vi "Error Name.vi"(10 "PCB LOCK":T1, 11 "Error Name":string[](array[string])=["Key Paid1(AI0)", "Key Paid1(AI1)", "Key Paid1(AI09)", "Key Paid1(AI10)", "Key Paid1(AI11)", "Key Paid1(AI12)"]) -> (3 "Error Message":string)   [LabVIEW 2015]
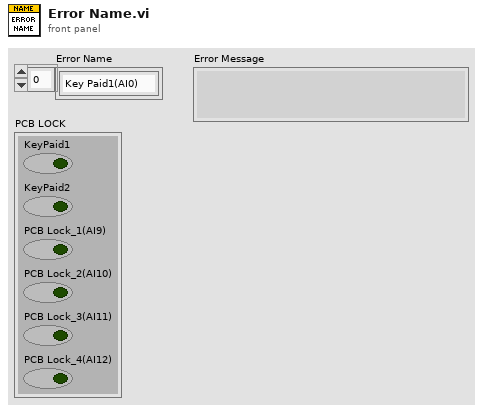
[diagram p1: front panel]
types:
  T1 = cluster{"KeyPaid1":bool, "KeyPaid2":bool, "PCB Lock_1(AI9)":bool, "PCB Lock_2(AI10)":bool, "PCB Lock_3(AI11)":bool, "PCB Lock_4(AI12)":bool}
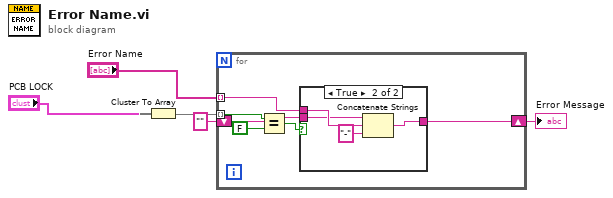
[diagram p0: block diagram]
diagram:
  n1 = Cluster To Array(cluster="PCB LOCK") -> (array=w2:bool[])
  n2 = for {
    tunnel: w2 -> [w11] mode=indexing
    tunnel: "Error Name" -> [w8] mode=indexing
    shift-right: [w7] -> w5
    shift-left: "" -> [w6]
    n3 = Equal?(x=w11, y=FALSE) -> (x = y?=w9:bool)
    n4 = case shown="True" w9 {
      tunnel: w8 -> [_ w16]
      tunnel: [w12 w15] -> w7
      tunnel: w6 -> [w12 w14]
      frame False {
      }
      frame True {
        n5 = Concatenate Strings(w14, w16, "-" ("string")) -> (w15:string)
      }
    }
  }
  "Error Message" <- w5
